vi "Set Column Color.vi"(8 "error in":errorcluster, 9 "color":u32(colorbox)=16777215, 10 "length":i32, 11 "XLS in":refnum<class "XLS.lvclass">) -> (0 "error out":errorcluster, 3 "XLS out":refnum<class "XLS.lvclass">)   [LabVIEW 2017, in "Report_lib.lvlib" / "XLS.lvclass"]
doc: "This method sett color of row\nwith certain length"
uses:
  XLS.lvclass
  XLS.lvclass/XLS.ctl
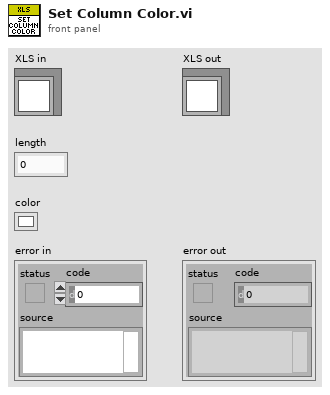
[diagram p1: front panel]
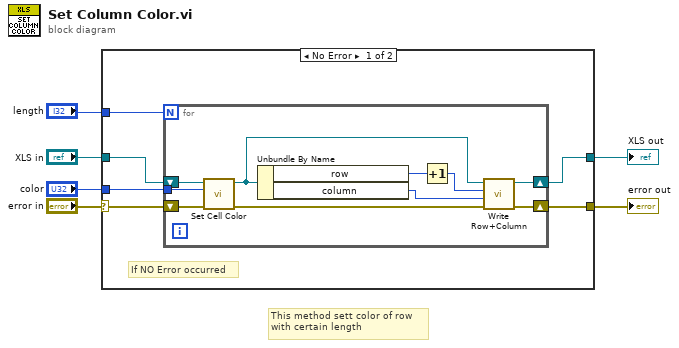
[diagram p0: block diagram]
diagram:
  # "This method sett color of row\nwith certain length"
  n1 = case shown="No Error" "error in" {
    selector: "error in" -> [w8 w24]
    tunnel: [w7 w24] -> w5
    tunnel: [w9 w23] -> w3
    tunnel: "XLS in" -> [w10 w23]
    tunnel: "length" -> [w12 _]
    tunnel: "color" -> [w11 _]
    frame No Error {
      # "If NO Error occurred"
      n2 = for {
        N: w12 -> [_]
        shift-right: [w19] -> w7
        shift-left: w8 -> [w21]
        shift-right: [w18] -> w9
        shift-left: w10 -> [w22]
        tunnel: w11 -> [w16]
        n3 = call "Set Cell Color.vi"("error in"=w21, "color"=w16, "XLS in"=w22) -> ("error out"=w20:errorcluster, "XLS out"=w17:refnum<class "XLS.lvclass">)  [unwired: 7 in]
        n4 = Unbundle By Name(w17) -> ("row"=w15:i32, "column"=w13:i32)
        n5 = Increment(x=w15) -> (x+1=w14:i32)
        n6 = call "Write Row+Column.vi"("error in"=w20, "column"=w13, "row"=w14, "XLS in"=w17) -> ("error out"=w19:errorcluster, "XLS out"=w18:refnum<class "XLS.lvclass">)  [unwired: 6 in]
      }
    }
    frame Error {
    }
  }
  "error out" <- w5
  "XLS out" <- w3
